vi "testErrorCode.vi"() -> ()   [LabVIEW 2019, in "ErrorTest.lvlib" / "ExpectationFailedError.lvlib"]
uses:
  ExpectationFailedError.lvlib
  Error/Error.lvlib
  Assertion/Assertion.lvlib
panel:
  out "error out":errorcluster
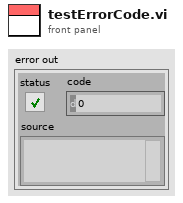
[diagram p1: front panel]
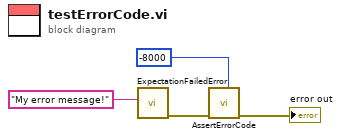
[diagram p0: block diagram]
diagram:
  n1 = call "ExpectationFailedError.vi"("Message"="My error message!") -> ("error out"=w4:errorcluster)  [unwired: 10 in]
  n2 = call "AssertErrorCode.vi"("Expected"=-8000, "error in (no error)"=w4) -> ("error out"=→"error out":errorcluster)  [unwired: 9 in]
